vi "ChannelsforTrigger.vi"(0 "Trigger":T1(ring)=enum."Line", 11 "error in":T3) -> (3 "SourceText_ChNum":cluster{"RingText.Text":string, i32}[](array[cluster])=[{"RingText.Text"="ADC 2", 0}, {"RingText.Text"="ADC 1", 1}], 4 "Corresponding channels":i32[](array[numeric])=[0, 1], 6 "Corresponding sources":i32[](array[numeric])=[1, 0], 8 "SourceText&RisingNum":cluster{"RingText.Text":string, i32}[](array[cluster])=[{"RingText.Text"="ADC 2", 0}, {"RingText.Text"="ADC 1", 1}], 10 "SourceText&Num":cluster{"RingText.Text":string, i32}[](array[cluster])=[{"RingText.Text"="ADC 2", 1}, {"RingText.Text"="ADC 1", 0}], 15 "error out":T3)   [LabVIEW 2016]
doc: "This VI gives you information about the channels. If you pass a trigger as input to the VI, you will get the following outputs:\n-sourceText_ChNum: This array of clusters contains the channel numbers which are triggered by the input \"Trigger\" as the second element of the cluster. The first element is the name of the source that is set for the channel.\n-Corresponding channels: This array of integer contains all channel numbers that are triggered by the input-trigger.\n-Corresponding sources: This array contains all source-numbers of the channels that are triggered by the input \"Trigger\".\n-SourceText&RisingNum: Array of clusters of two elements. It contains the set source for the input \"Trigger\". The second element is a number that equals the array index of the array of clusters.\n-SourceText&Num: This array of clusters of two elements contains the set source for the input \"Trigger\". The second element is the corresponding number of the source as it is defined in the typedef \"channel-source_selection\"."
uses:
  Controls/Error_Out.ctl
  Controls/Channel-Source_Selection.ctl
panel:
  out "Source 2":T2 items=["[read only]"=-2147483648, "ADC 1"=0, "ADC 2"=1, "ADC 3"=2, "ADC 4"=3, "ADC 5"=4, "ADC 6"=5, "HF 1 Out"=7, "HF 1 df"=8, "z out"=9, "HF 1"=12, "HF 1 Ampl."=13, "HF 1 Phase"=14, "LF LockIn Ampl"=16, "LF LockIn Phase"=17, "z out inv"=18, "counter"=23, "Crosslink 1"=29, "Crosslink 2"=30, "Pos X"=31, "Pos Y"=32]
  in  "Stop Button":bool
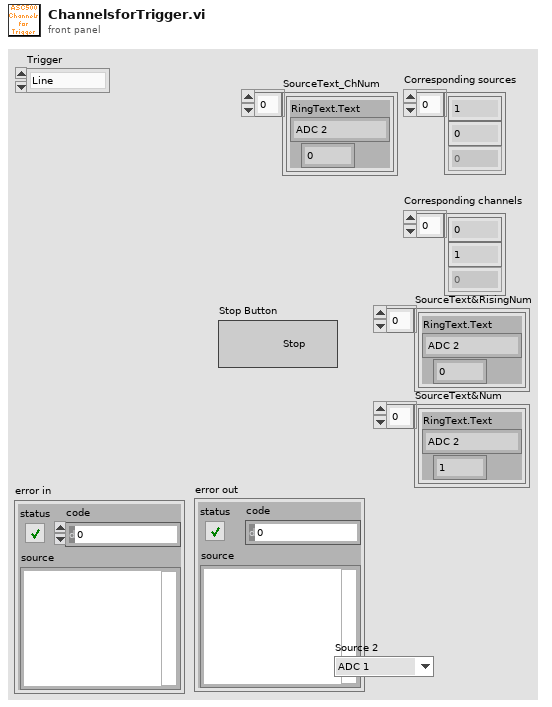
[diagram p1: front panel]
types:
  T1 = enum32{"Disabled", "Scan", "Line", "Spec 1", "Spec 2", "Spec 3", "Cal", "Trigger", "Every", "SoftSpec", "DualPass", "Step Scan"}
  T2 = typedef "Channel-Source_Selection.ctl" = i32
  T3 = typedef "Error_Out.ctl" = errorcluster
  T4 = enum16{"Input", "checkCH", "display disabled", "which source", "Abort"}
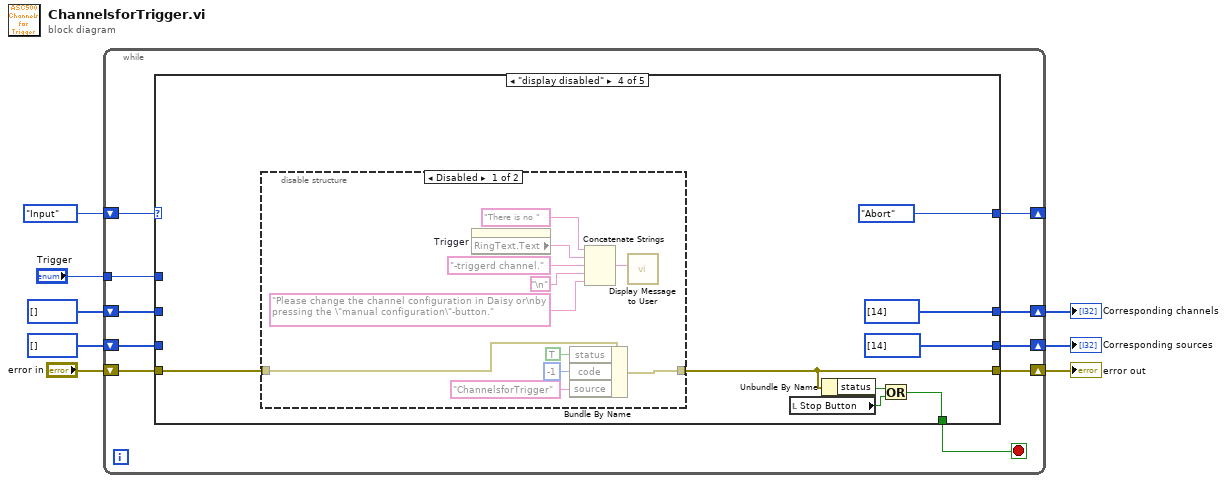
[diagram p0: block diagram]
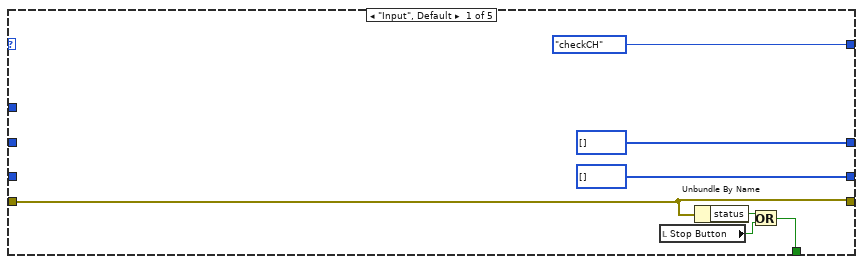
[diagram p2: hidden frame]
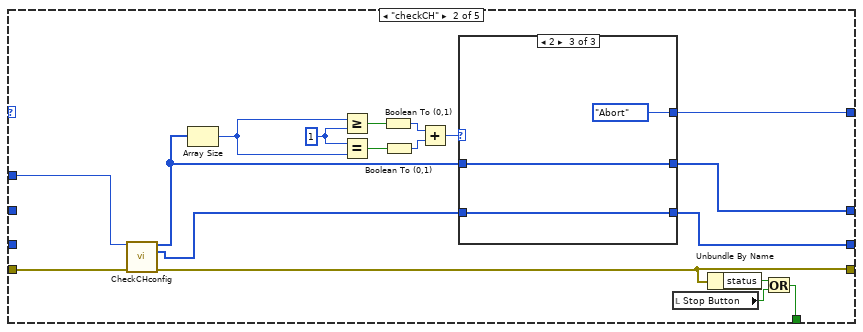
[diagram p3: hidden frame]
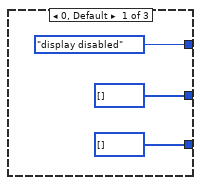
[diagram p4: hidden frame]
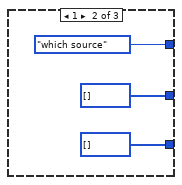
[diagram p5: hidden frame]
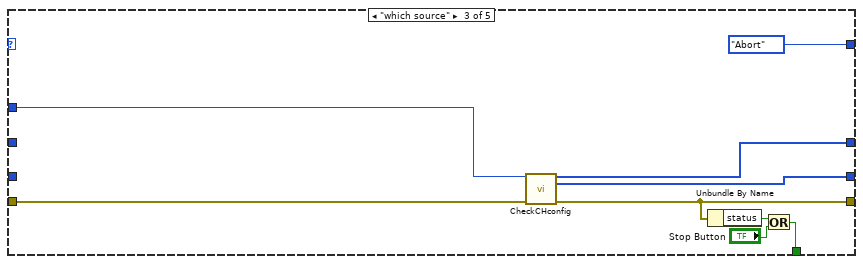
[diagram p6: hidden frame]
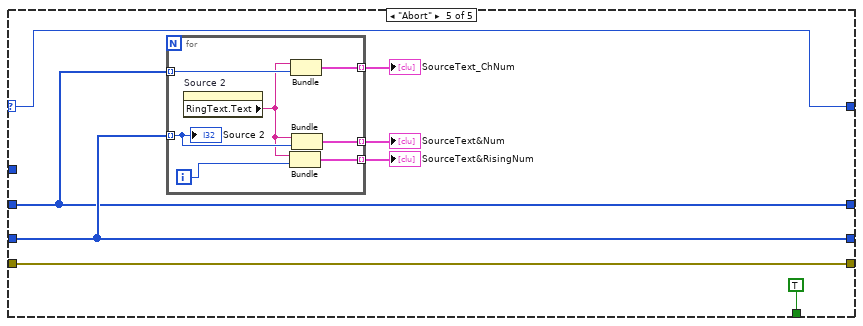
[diagram p8: hidden frame]
diagram:
  n1 = while {
    shift-right: [w17] -> w7
    shift-left: "error in" -> [w18]
    shift-right: [w16] -> w4
    shift-left: i32[] [] -> [w15]
    shift-right: [w14] -> w3
    shift-left: i32[] [] -> [w13]
    shift-right: [w11] -> _
    shift-left: T4."Input" ("State") -> [w12]
    tunnel: "Trigger" -> [w9]
    stop <- w10 stop-if-true
    n2 = case shown="\"display disabled\"" w12 {
      selector: w12 -> [_ _ _ _ w82]
      tunnel: w18 -> [w25 w43 w58 w62 w89]
      tunnel: [w25 w34 w57 w63 w89] -> w17
      tunnel: [w21 w31 w60 w66 TRUE] -> w10
      tunnel: [i32[] [] ("Corresponding channels") w30 w56 i32[] [14] ("Corresponding channels") w84] -> w16
      tunnel: w15 -> [_ _ _ _ w84]
      tunnel: [i32[] [] ("Corresponding channels") w29 w53 i32[] [14] ("Corresponding channels") w86] -> w14
      tunnel: w13 -> [_ _ _ _ w86]
      tunnel: [T4."checkCH" ("State") w28 T4."Abort" ("State") T4."Abort" ("State") w82] -> w11
      tunnel: w9 -> [_ w27 w54 _ _]
      frame "Input", Default {
        n3 = local read "Stop Button"() -> (w23:bool)
        n4 = Unbundle By Name(w25) -> ("status"=w24:bool)
        n5 = Or(x=w24, y=w23) -> (x .or. y?=w21:bool)
      }
      frame "checkCH" {
        w41 = 1 ("y")
        n6 = call "CheckCHconfig.vi"("Trigger"=w27, "error in"=w43) -> ("Corresponding channels"=w32:i32[], "Corresponding trig_sources"=w26:i32[], "error out"=w34:T3)  [unwired: 10 in, 1 out]
        n7 = Array Size(array=w32) -> (size(s)=w42:i32)
        n8 = Greater Or Equal?(x=w42, y=w41) -> (x >= y?=w40:bool)
        n9 = Equal?(x=w41, y=w42) -> (x = y?=w39:bool)
        n10 = Boolean To (0,1)(Boolean=w40) -> (0, 1=w38:i16)
        n11 = Boolean To (0,1)(Boolean=w39) -> (0, 1=w36:i16)
        n12 = Add(x=w38, y=w36) -> (x+y=w37:i16)
        n13 = case shown="2" w37 {
          tunnel: w32 -> [_ _ w52]
          tunnel: [T4."display disabled" ("State") T4."which source" ("State") T4."Abort" ("State")] -> w28
          tunnel: w26 -> [_ _ w51]
          tunnel: [i32[] [] ("Corresponding channels") i32[] [] ("Corresponding channels") w52] -> w30
          tunnel: [i32[] [] ("Corresponding channels") i32[] [] ("Corresponding channels") w51] -> w29
          frame 0, Default {
          }
          frame 1 {
          }
          frame 2 {
          }
        }
        n14 = local read "Stop Button"() -> (w33:bool)
        n15 = Unbundle By Name(w34) -> ("status"=w35:bool)
        n16 = Or(x=w35, y=w33) -> (x .or. y?=w31:bool)
      }
      frame "which source" {
        n17 = call "CheckCHconfig.vi"("Trigger"=w54, "error in"=w58) -> ("Corresponding channels"=w56:i32[], "Corresponding trig_sources"=w53:i32[], "error out"=w57:T3)  [unwired: 10 in, 1 out]
        n18 = Unbundle By Name(w57) -> ("status"=w61:bool)
        n19 = Or(x=w61, y="Stop Button") -> (x .or. y?=w60:bool)
      }
      frame "display disabled" {
        n20 = disable-structure shown="Disabled" {
          disable-tunnel: [w74 w81] -> w63
          disable-tunnel: w62 -> [w73 w81]
          frame Disabled {
            n21 = property on="Trigger" class="Enum (strikt)"() -> ("RingText.Text"=w76:string)  [unwired: 2 in, 2 out]
            n22 = Bundle By Name(cluster=w73, "status"=TRUE, "code"=-1, "source"="ChannelsforTrigger") -> (w74:T3)
            n23 = Concatenate Strings("There is no " ("Message"), w76, "-triggerd channel." ("Message"), "\n", "Please change the channel configuration in Daisy or\nby pressing the \"manual configuration\"-button." ("Message")) -> (w77:string)
            n24 = call "Display Message to User"("Message"=w77) -> ()  [unwired: 9 in, 2 out]
          }
          frame Enabled {
          }
        }
        n25 = local read "Stop Button"() -> (w68:bool)
        n26 = Unbundle By Name(w63) -> ("status"=w69:bool)
        n27 = Or(x=w69, y=w68) -> (x .or. y?=w66:bool)
      }
      frame "Abort" {
        n28 = for {
          tunnel: w86 -> [w96] mode=indexing
          tunnel: [w95] -> w87 mode=indexing
          tunnel: w84 -> [w93] mode=indexing
          tunnel: [w94] -> w85 mode=indexing
          tunnel: [w90] -> w83 mode=indexing
          i -> [w91]
          n29 = property on="Source 2" class="Ring (strikt)"() -> ("RingText.Text"=w92:string)  [unwired: 2 in, 2 out]
          n30 = Bundle("RingText.Text"=w92, w91) -> (w90:cluster{"RingText.Text":string, i32})  [unwired: 1 in]
          n31 = Bundle("RingText.Text"=w92, w93) -> (w94:cluster{"RingText.Text":string, i32})  [unwired: 1 in]
          n32 = Bundle("RingText.Text"=w92, w96) -> (w95:cluster{"RingText.Text":string, i32})  [unwired: 1 in]
          "Source 2" <- w96
        }
        "SourceText&Num" <- w87
        "SourceText_ChNum" <- w85
        "SourceText&RisingNum" <- w83
      }
    }
  }
  "error out" <- w7
  "Corresponding channels" <- w4
  "Corresponding sources" <- w3
